vi "AVQ8347 Center Center.vi"(8 "Error In":errorcluster, 9 "Center Point Unit (nm)":enum16{"um", "nm", "THz", "GHz"}(ring)=enum."nm", 10 "Center Point Value (700)":dbl=700.0 format="%.2f", 11 "VISA Session":refnum<visa-resource-name>) -> (0 "Error Out":errorcluster, 2 "Send Code":string, 3 "Copy VISA Session":refnum<visa-resource-name>)   [LabVIEW 2021]
doc: "Setting of analysis center wavelength"
panel:
  # "Center Center"
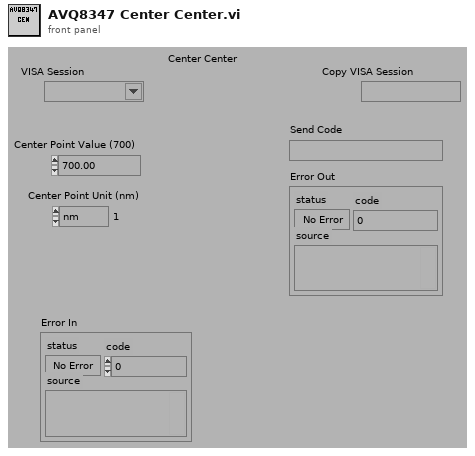
[diagram p1: front panel]
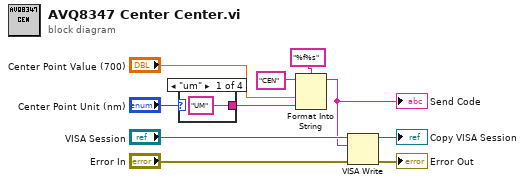
[diagram p0: block diagram]
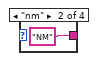
[diagram p2: hidden frame]
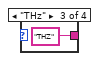
[diagram p3: hidden frame]
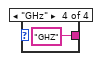
[diagram p4: hidden frame]
diagram:
  n1 = case shown="\"um\"" "Center Point Unit (nm)" {
    tunnel: ["UM" "NM" "THZ" "GHZ"] -> w1
    frame "um" {
    }
    frame "nm" {
    }
    frame "THz" {
    }
    frame "GHz" {
    }
  }
  n2 = Format Into String(format string="%f%s", initial string="CEN", "Center Point Value (700)", w1) -> (resulting string=w2:string)  [unwired: 1 in, 1 out]
  "Send Code" <- w2
  n3 = VISA Write(VISA resource name="VISA Session", write buffer=w2, error in (no error)="Error In") -> (VISA resource name out=→"Copy VISA Session":refnum<visa-resource-name>, error out=→"Error Out":errorcluster)  [unwired: 1 out]
